vi "Move command constructor.vi"(4 "Z Limit (+/- um)":sgl, 6 "Z Current":sgl, 7 "Bypass Z-safety interlock":bool, 8 "error in (no error)":errorcluster, 9 "Z":sgl, 10 "Y":sgl, 11 "X":sgl) -> (0 "error out":errorcluster, 1 "Adjusted Z":sgl, 2 "Adjusted Y":sgl, 3 "Move command":string, 5 "Adjusted X":sgl)   [LabVIEW 2020, in "TranslationStageClassStructure.lvlib" / "Scientifica XYZ Gen1.lvclass"]
uses:
  Scientifica XYZ Gen1.lvclass
  Typedefs/Z intelock check type.ctl
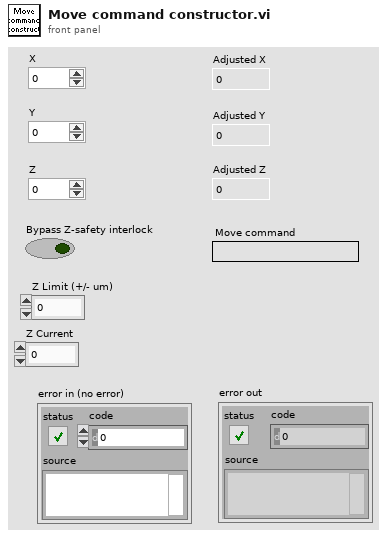
[diagram p1: front panel]
types:
  T1 = typedef "Z intelock check type.ctl" = enum16{"Check against Z limit", "Check againt current position"}
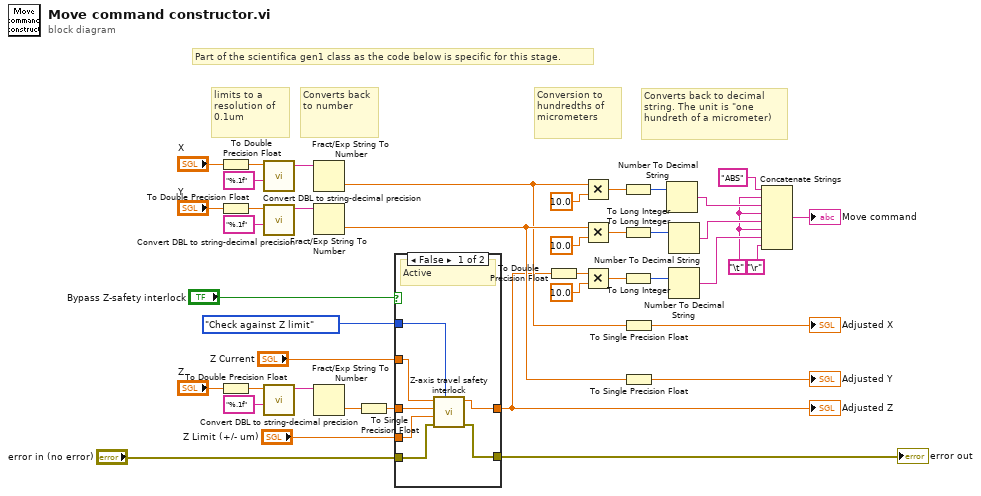
[diagram p0: block diagram]
diagram:
  w22 = "\t" ("Tab Constant")
  # "Part of the scientifica gen1 class as the code below is specific for this stage."
  # "Converts back to decimal string. The unit is \"one hundreth of a micrometer)"
  # "Converts back to number"
  # "limits to a resolution of 0.1um"
  # "Conversion to hundredths of micrometers"
  n1 = To Double Precision Float(number="X") -> (double precision float=w9:dbl)
  n2 = To Double Precision Float(number="Y") -> (double precision float=w8:dbl)
  n3 = To Double Precision Float(number="Z") -> (double precision float=w7:dbl)
  n4 = call <userlib>:"Convert DBL to string-decimal precision.vi"("Format (%f)"="%.1f", "DBL Value"=w9) -> ("Converted to String"=w33:string)  [unwired: 9 in]
  n5 = call <userlib>:"Convert DBL to string-decimal precision.vi"("Format (%f)"="%.1f", "DBL Value"=w8) -> ("Converted to String"=w34:string)  [unwired: 9 in]
  n6 = call <userlib>:"Convert DBL to string-decimal precision.vi"("Format (%f)"="%.1f", "DBL Value"=w7) -> ("Converted to String"=w35:string)  [unwired: 9 in]
  n7 = Fract/Exp String To Number(string=w33) -> (number=w41:dbl)  [unwired: 3 in, 1 out]
  n8 = Fract/Exp String To Number(string=w34) -> (number=w42:dbl)  [unwired: 3 in, 1 out]
  n9 = Fract/Exp String To Number(string=w35) -> (number=w13:dbl)  [unwired: 3 in, 1 out]
  n10 = To Single Precision Float(number=w13) -> (single precision float=w11:sgl)
  n11 = case shown="False" "Bypass Z-safety interlock" {
    tunnel: [w49 w51] -> w12
    tunnel: w11 -> [w48 w51]
    tunnel: Z_intelock_check_type."Check against Z limit" ("Interlock check type") -> [w47 _]
    tunnel: "Z Limit (+/- um)" -> [w46 _]
    tunnel: "Z Current" -> [w45 _]
    tunnel: "error in (no error)" -> [w44 w50]
    tunnel: [w43 w50] -> w1
    frame False {
      # "Active"
      n12 = call "Z-axis travel safety interlock.vi"("Interlock check type"=w47, "error in (no error)"=w44, "Z Limit (+/- um)"=w46, "Z move to"=w48, "Z Current"=w45) -> ("error out"=w43:errorcluster, "Z"=w49:sgl)  [unwired: 5 in]
    }
    frame True {
      # "Bypassed"
    }
  }
  "Adjusted Z" <- w12
  "error out" <- w1
  n13 = To Double Precision Float(number=w12) -> (double precision float=w10:dbl)
  n14 = Multiply(x=w41, y=10.0) -> (x*y=w17:dbl)
  n15 = Multiply(x=w42, y=10.0) -> (x*y=w37:dbl)
  n16 = Multiply(x=w10, y=10.0) -> (x*y=w39:dbl)
  n17 = To Long Integer(number=w17) -> (32bit integer=w16:i32)
  n18 = To Long Integer(number=w37) -> (32bit integer=w15:i32)
  n19 = To Long Integer(number=w39) -> (32bit integer=w14:i32)
  n20 = To Single Precision Float(number=w41) -> (single precision float=→"Adjusted X":sgl)
  n21 = To Single Precision Float(number=w42) -> (single precision float=→"Adjusted Y":sgl)
  n22 = Number To Decimal String(number=w16) -> (decimal integer string=w36:string)  [unwired: 1 in]
  n23 = Number To Decimal String(number=w15) -> (decimal integer string=w38:string)  [unwired: 1 in]
  n24 = Number To Decimal String(number=w14) -> (decimal integer string=w40:string)  [unwired: 1 in]
  n25 = Concatenate Strings("ABS" ("decimal integer string"), w22, w36, w22, w38, w22, w40, "\r" ("Carriage Return Constant")) -> (→"Move command":string)
